vi "CycleRenameGroup.vi"(11 "TreeControl输入":refnum<vi>) -> (0 "更新后的组名":string, 3 "行索引":i32)   [LabVIEW 2020, in "Curve Editor.lvlib"]
uses:
  Curve Editor.lvlib
panel:
  # "对树形选中的组标识进行重命名，并返回更新后的组名及行索引"
  # "其功能已被EditGroup取代"
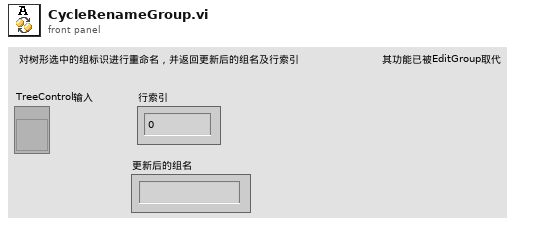
[diagram p1: front panel]
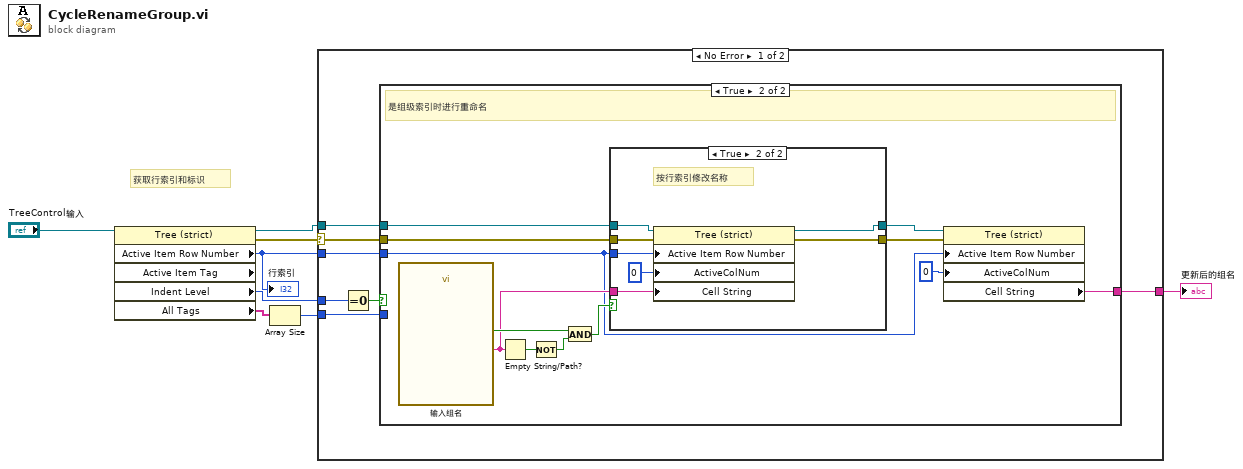
[diagram p0: block diagram]
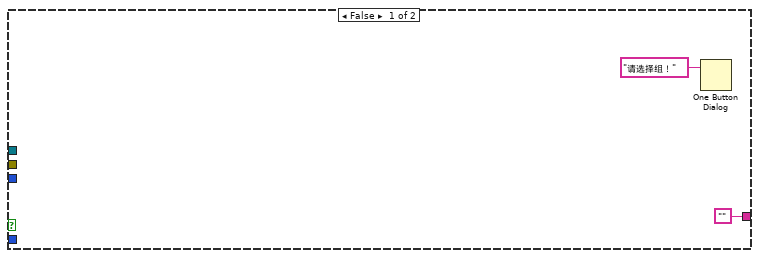
[diagram p2: hidden frame]
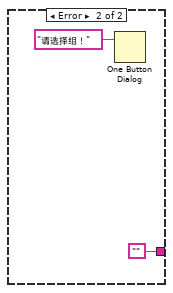
[diagram p4: hidden frame]
diagram:
  # "获取行索引和标识"
  n1 = property class="Tree (strict)" props=["Active Item Row Number", "Active Item Tag", "Indent Level", "All Tags"](reference="TreeControl输入") -> (reference out=w5:refnum<vi>, error out=w6:errorcluster, "Active Item Row Number"=w2:i32, "Indent Level"=w4:i32, "All Tags"=w7:string[])  [unwired: 1 in, 1 out]
  "行索引" <- w2
  n2 = Array Size(array=w7) -> (size(s)=w8:i32)
  n3 = case shown="No Error" w6 {
    selector: w6 -> [w13 _]
    tunnel: w4 -> [w15 _]
    tunnel: w5 -> [w11 _]
    tunnel: w8 -> [w12 _]
    tunnel: w2 -> [w10 _]
    tunnel: [w9 ""] -> w1
    frame No Error {
      n4 = Equal To 0?(x=w15) -> (x = 0?=w14:bool)
      n5 = case shown="True" w14 {
        tunnel: w11 -> [_ w29]
        tunnel: w13 -> [_ w28]
        tunnel: w12 -> [_ _]
        tunnel: w10 -> [_ w20]
        tunnel: ["" w21] -> w9
        frame False {
          n6 = One Button Dialog(message="请选择组！" ("消息")) -> ()  [unwired: 1 in, 1 out]
        }
        frame True {
          # "是组级索引时进行重命名"
          n7 = call "输入组名"() -> ("新组名"=w23:string, "确定"=w25:bool)  [unwired: 17 in, 1 out]
          n8 = Empty String/Path?(string/path=w23) -> (empty?=w27:bool)
          n9 = Not(x=w27) -> (.not. x?=w26:bool)
          n10 = And(x=w25, y=w26) -> (x .and. y?=w24:bool)
          n11 = case shown="True" w24 {
            tunnel: w29 -> [w31 w38]
            tunnel: w28 -> [w30 w37]
            tunnel: w20 -> [_ w36]
            tunnel: w23 -> [_ w35]
            tunnel: [w31 w34] -> w22
            tunnel: [w30 w33] -> w19
            frame False {
            }
            frame True {
              # "按行索引修改名称"
              n12 = property class="Tree (strict)"(reference=w38, error in=w37, "Active Item Row Number"=w36, "ActiveColNum"=0 ("活动单元格:活动列数"), "Cell String"=w35) -> (reference out=w34:refnum<vi>, error out=w33:errorcluster)
            }
          }
          n13 = property class="Tree (strict)"(reference=w22, error in=w19, "Active Item Row Number"=w20, "ActiveColNum"=0 ("活动单元格:活动列数")) -> ("Cell String"=w21:string)  [unwired: 2 out]
        }
      }
    }
    frame Error {
      n14 = One Button Dialog(message="请选择组！" ("消息")) -> ()  [unwired: 1 in, 1 out]
    }
  }
  "更新后的组名" <- w1
